vi "Configure Cameras.vi"(8 "error in (no error)":errorcluster, 11 "Gantry Class in":refnum<class "Gantry Class.lvclass">) -> (0 "error out":errorcluster, 3 "Gantry Class out":refnum<class "Gantry Class.lvclass">)   [LabVIEW 2011, in "Gantry Class.lvclass"]
uses:
  Gantry Class.lvclass
  <vilib>/userdefined/High Color/IMAQdx.ctl
  <vilib>/vision/driver/NI_Vision_Acquisition_Software.lvlib
panel:
  in  "Camera":cluster{"Name":string, "IMAQ Session":T1}
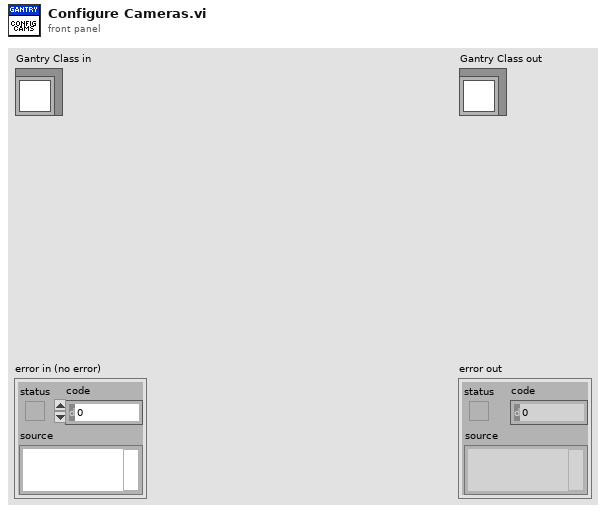
[diagram p1: front panel]
types:
  T1 = typedef "IMAQdx.ctl" = refnum<k21>
  T2 = cluster{"Type":u32, "Version":u32, "Flags":u32, "SerialNumberHigh":u32, "SerialNumberLow":u32, "BusType":u32, "InterfaceName":string, "VendorName":string, "ModelName":string, "CameraFileName":string, "CameraAttributeURL":string}[]
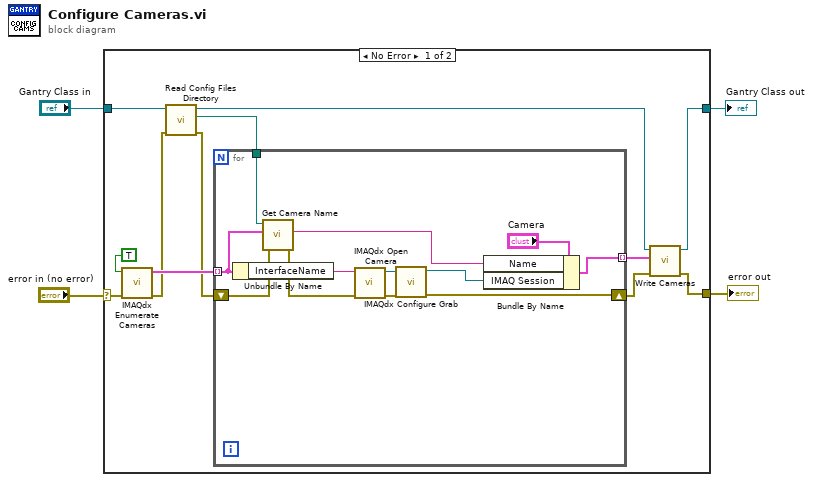
[diagram p0: block diagram]
diagram:
  n1 = case shown="No Error" "error in (no error)" {
    selector: "error in (no error)" -> [w11 w30]
    tunnel: [w10 w30] -> w3
    tunnel: [w13 w29] -> w1
    tunnel: "Gantry Class in" -> [w7 w29]
    frame No Error {
      n2 = call <vilib>:"IMAQdx Enumerate Cameras.vi"("error in"=w11, "Connected Only? (Yes)"=TRUE) -> ("error out"=w9:errorcluster, "Camera Information Array"=w15:T2)  [unwired: 8 in]
      n3 = call-dynamic "Read Config Files Directory.vi"("error in (no error)"=w9, "Gantry Class in"=w7) -> ("error out"=w8:errorcluster, "Config Files Directory"=w5:path, "Gantry Class out"=w6:refnum<class "Gantry Class.lvclass">)  [unwired: 7 in]
      n4 = for {
        tunnel: w15 -> [w21] mode=indexing
        tunnel: [w26] -> w14 mode=indexing
        shift-right: [w23] -> w12
        shift-left: w8 -> [w18]
        tunnel: w5 -> [w20]
        n5 = Unbundle By Name(w21) -> ("InterfaceName"=w27:string)
        n6 = call "Get Camera Name.vi"("error in (no error)"=w18, "IMAQdx Data"=w21, "Config File Directory"=w20) -> ("error out"=w17:errorcluster, "Camera Name"=w19:string)  [unwired: 7 in]
        n7 = call <vilib>:"IMAQdx Open Camera.vi"("error in"=w17, "Session In"=w27) -> ("error out"=w24:errorcluster, "Session Out"=w25:T1)  [unwired: 8 in]
        n8 = call <vilib>:"IMAQdx Configure Grab.vi"("error in"=w24, "Session In"=w25) -> ("error out"=w23:errorcluster, "Session Out"=w22:T1)  [unwired: 8 in]
        n9 = Bundle By Name(cluster="Camera", "Name"=w19, "IMAQ Session"=w22) -> (w26:cluster{"Name":string, "IMAQ Session":T1})
      }
      n10 = call-dynamic "Write Cameras.vi"("error in (no error)"=w12, "Cameras"=w14, "Gantry Class in"=w6) -> ("error out"=w10:errorcluster, "Gantry Class out"=w13:refnum<class "Gantry Class.lvclass">)  [unwired: 7 in]
    }
    frame Error {
    }
  }
  "error out" <- w3
  "Gantry Class out" <- w1
